vi "invokerunvi.vi"   [LabVIEW 2014]
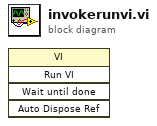
[diagram p0: block diagram]
diagram:
  n1 = invoke class="VI" method="Run VI"() -> ()  [unwired: 5 in, 5 out]
